vi "Resolve.vi"(8 "error in (no error)":errorcluster, 10 "Result":T1, 11 "Result in":refnum<class "Result.lvclass">) -> (0 "error out":errorcluster, 1 "Promise Already Resolved":bool, 2 "Future Already Completed":bool)   [LabVIEW 2017, in "Futures.lvlib" / "Result.lvclass"]
doc: "Resolves the result with an error cluster."
uses:
  Result.lvclass
  Result Data.ctl
  Result.lvclass/Result.ctl
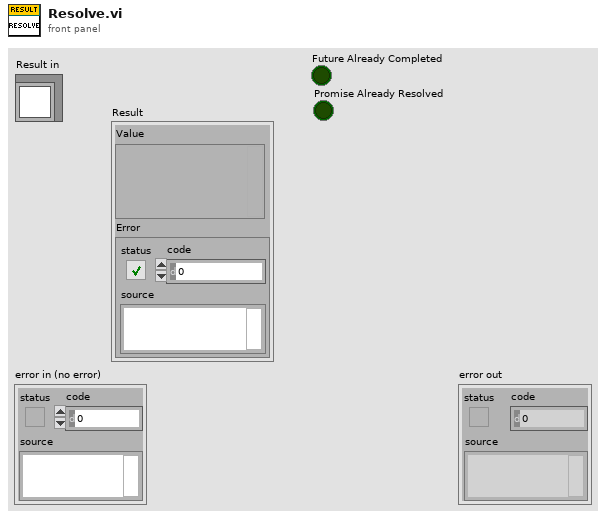
[diagram p1: front panel]
types:
  T1 = typedef "Futures.lvlib/Result.lvclass/Result Data.ctl" = cluster{"Value":variant, "Error":errorcluster}
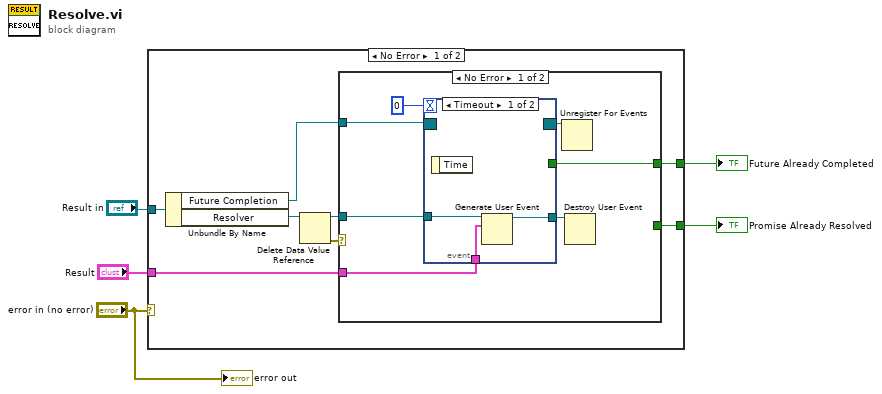
[diagram p0: block diagram]
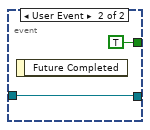
[diagram p2: hidden frame]
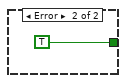
[diagram p3: hidden frame]
diagram:
  n1 = case shown="No Error" "error in (no error)" {
    tunnel: "Result in" -> [w13 _]
    tunnel: [w8 _] -> w3
    tunnel: [w7 _] -> w2
    tunnel: "Result" -> [w6 _]
    frame No Error {
      n2 = Unbundle By Name(w13) -> ("Future Completion"=w9:refnum<event-registration>, "Resolver"=w12:refnum<data-value>)
      n3 = Delete Data Value Reference(data value reference=w12) -> (data value=w10:refnum<user-event>, error out=w11:errorcluster)  [unwired: 1 in]
      n4 = case shown="No Error" w11 {
        tunnel: w10 -> [w16 _]
        tunnel: w9 -> [w20 _]
        tunnel: [w17 _] -> w8
        tunnel: [_ TRUE] -> w7
        tunnel: w6 -> [w14 _]
        frame No Error {
          n5 = event shown="[0] Timeout" {
            selector: w20 -> [_ _]
            dyn-events: [_ _] -> w18
            timeout: 0 -> [_ _]
            tunnel: [_ TRUE] -> w17
            tunnel: w16 -> [w23 w24]
            tunnel: [w22 w24] -> w15
            tunnel: w14 -> [w21 _]
            event Timeout {
              n6 = event-data() -> ()  [unwired: 1 in, 1 out]
              n7 = Generate User Event(user event=w23, event data cluster=w21) -> (user event out=w22:refnum<user-event>)  [unwired: 2 in, 1 out]
            }
            event User Event {
              n8 = event-data() -> ()  [unwired: 1 in, 1 out]
            }
          }
          n9 = Unregister For Events(event registration refnum=w18) -> ()  [unwired: 1 in, 1 out]
          n10 = Destroy User Event(user event=w15) -> ()  [unwired: 1 in, 1 out]
        }
        frame Error {
        }
      }
    }
    frame Error {
    }
  }
  "Future Already Completed" <- w3
  "Promise Already Resolved" <- w2
  "error out" <- "error in (no error)"
